vi "4 Edge Rake.vi"(2 "input cluster":errorcluster, 3 "Image Dst Out":T1) -> (0 "B":cluster{sgl, sgl, sgl, sgl}, 1 "M":cluster{sgl, sgl, sgl, sgl})   [LabVIEW 2011]
uses:
  <vilib>/vision/Image Controls.llb/IMAQ Image.ctl
  <vilib>/vision/NI_Vision_Development_Module.lvlib
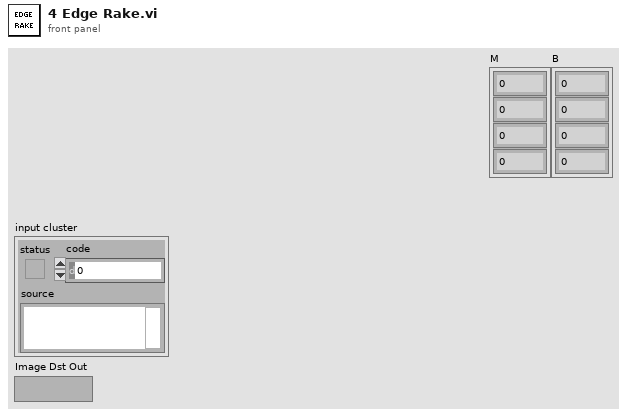
[diagram p1: front panel]
types:
  T1 = typedef "IMAQ Image.ctl" = refnum<image>
  T2 = cluster{"Show Search Area":bool, "Show Search Lines":bool, "Show Edges Found":bool, "Show Result":bool}
  T3 = cluster{"Number of Lines":i32, "Type":enum32{"First Edge Rake", "Best Edge Rake", "Hough Edge Rake", "First Edge Projection", "Best Edge Projection"}, "Min. Score":dbl, "Max. Score":dbl, "Orientation":dbl, "Angle Range":dbl, "Angle Tolerance":dbl, "Step Size":u32, "Min. SNR (db)":dbl, "Min. Points (%)":dbl, "Hough Iterations":i32}
  T4 = cluster{"Edge Polarity":u32, "Kernel Size":u32, "Width":u32, "Minimum Edge Strength":sgl, "Interpolation Type":enum32{"Zero Order", "Bilinear", "Quadratic", "Cubic", "Bilinear Fixed"}, "Data Processing Method":enum32{"Average", "Median"}}
  T5 = cluster{"Global Rectangle":i32[], "Contours":cluster{"ID":enum32{"External", "Internal"}, "Type":u32, "Coordinates":i32[]}[]}
  T6 = cluster{"Point1 (Pixels)":cluster{"X":sgl, "Y":sgl}, "Point2 (Pixels)":cluster{"X":sgl, "Y":sgl}, "Point1 (Real-World)":cluster{"X":sgl, "Y":sgl}, "Point2 (Real-World)":cluster{"X":sgl, "Y":sgl}, "Angle (Pixel)":dbl, "Angle (Real-World)":dbl, "Score":dbl, "Straightness":dbl, "Average SNR (db)":dbl, "Calibration Valid":bool}[]
  T7 = typedef "Search Line.ctl" = cluster{"Start Point":cluster{"X":sgl, "Y":sgl}, "End Point":cluster{"X":sgl, "Y":sgl}, "Edge Info":T8[], "Edge Map":dbl[], "Calibration Valid":bool}
  T8 = typedef "Edge New.ctl" = cluster{"Location (Pixel)":cluster{"X":sgl, "Y":sgl}, "Location (Real-World)":cluster{"X":sgl, "Y":sgl}, "Distance (Pixel)":dbl, "Distance (Real-World)":dbl, "Strength":dbl, "Noise":dbl, "Rising?":bool}
  T9 = cluster{"Straight Edges":cluster{"Point1 (Pixels)":cluster{"X":sgl, "Y":sgl}, "Point2 (Pixels)":cluster{"X":sgl, "Y":sgl}, "Point1 (Real-World)":cluster{"X":sgl, "Y":sgl}, "Point2 (Real-World)":cluster{"X":sgl, "Y":sgl}, "Angle (Pixel)":dbl, "Angle (Real-World)":dbl, "Score":dbl, "Straightness":dbl, "Average SNR (db)":dbl, "Calibration Valid":bool}[], "Search Lines Information":T7[], "Used Edges":cluster{"Edge Information":T8[]}[]}
  T10 = cluster{"Point1 (Pixels)":cluster{"X":sgl, "Y":sgl}, "Point2 (Pixels)":cluster{"X":sgl, "Y":sgl}, "Point1 (Real-World)":cluster{"X":sgl, "Y":sgl}, "Point2 (Real-World)":cluster{"X":sgl, "Y":sgl}, "Angle (Pixel)":dbl, "Angle (Real-World)":dbl, "Score":dbl, "Straightness":dbl, "Average SNR (db)":dbl, "Calibration Valid":bool}
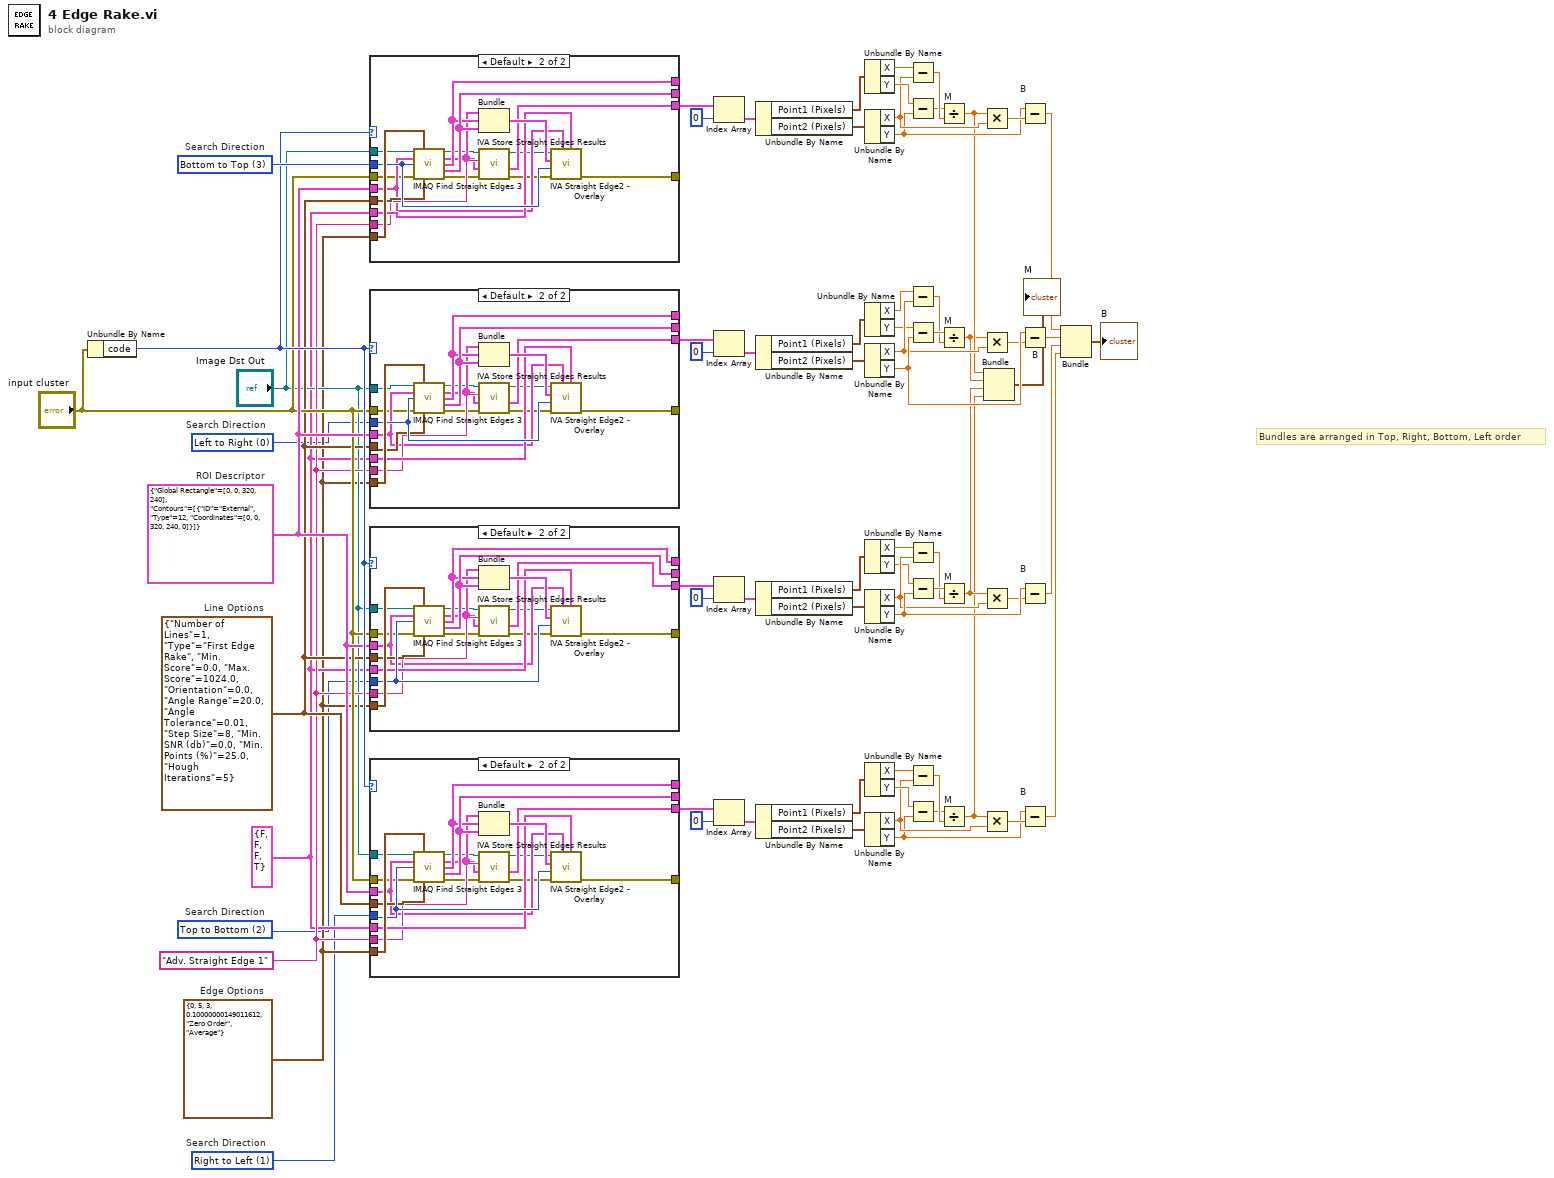
[diagram p0: block diagram]
diagram:
  w54 = u32 1 items=["Left to Right", "Right to Left", "Top to Bottom", "Bottom to Top"]  # Search Direction
  w56 = u32 2 items=["Left to Right", "Right to Left", "Top to Bottom", "Bottom to Top"]  # Search Direction
  w55 = u32 0 items=["Left to Right", "Right to Left", "Top to Bottom", "Bottom to Top"]  # Search Direction
  w60 = "Adv. Straight Edge 1" ("Step Name")
  w58 = T2 {"Show Search Area"=FALSE, "Show Search Lines"=FALSE, "Show Edges Found"=FALSE, "Show Result"=TRUE} ("Setup")
  w61 = T3 {"Number of Lines"=1, "Type"=enum."First Edge Rake", "Min. Score"=0.0, "Max. Score"=1024.0, "Orientation"=0.0, "Angle Range"=20.0, "Angle Tolerance"=0.01, "Step Size"=8, "Min. SNR (db)"=0.0, "Min. Points (%)"=25.0, "Hough Iterations"=5}  # Line Options
  w70 = u32 3 items=["Left to Right", "Right to Left", "Top to Bottom", "Bottom to Top"]  # Search Direction
  w57 = T4 {"Edge Polarity"=0, "Kernel Size"=5, "Width"=3, "Minimum Edge Strength"=0.1, "Interpolation Type"=enum."Zero Order", "Data Processing Method"=enum."Average"}  # Edge Options
  w63 = T5 {"Global Rectangle"=[0, 0, 320, 240], "Contours"=[{"ID"=enum."External", "Type"=12, "Coordinates"=[0, 0, 320, 240, 0]}]}  # ROI Descriptor
  # "Bundles are arranged in Top, Right, Bottom, Left order"
  n1 = Unbundle By Name("input cluster") -> ("code"=w64:i32)
  n2 = case shown="Default" w64 {
    tunnel: w57 -> [_ w88]
    tunnel: w70 -> [_ w87]
    tunnel: w61 -> [_ w86]
    tunnel: [_ w84] -> _
    tunnel: w58 -> [_ w83]
    tunnel: [_ w82] -> _
    tunnel: [_ w81] -> _
    tunnel: w60 -> [_ w80]
    tunnel: [_ w79] -> w65
    tunnel: w63 -> [_ w77]
    tunnel: "input cluster" -> [_ w72]
    tunnel: "Image Dst Out" -> [_ w71]
    frame -1074396199, -1074396198 {
      # "Discard Coordinate System Error"
    }
    frame Default {
      n3 = call "IMAQ Find Straight Edges 3"("Image"=w71, "Edge Options"=w88, "ROI Descriptor"=w77, "Search Direction"=w87, "error in (no error)"=w72, "Line Options"=w86) -> ("Image (duplicate)"=w76:T1, "Straight Edges"=w78:T6, "Search Lines Information"=w81:T7[], "Used Edges"=w82:cluster{"Edge Information":T8[]}[], "error out"=w74:errorcluster)  [unwired: 1 in, 4 out]
      n4 = Bundle("Straight Edges"=w78, "Search Lines Information"=w81, "Used Edges"=w82) -> (w85:T9)  [unwired: 1 out]
      n5 = call <vilib>:"IVA Store Straight Edges Results.vi"("error in (no error)"=w74, "Straight Edges"=w78, "Step Name"=w80, "Image in"=w76) -> ("error out"=w73:errorcluster, "Straight Edges dup"=w79:T6, "Image dup"=w75:T1)  [unwired: 5 out]
      n6 = call <vilib>:"IVA Straight Edge2 - Overlay.vi"("Setup"=w83, "Search Area"=w77, "error in (no error)"=w73, "Scan Direction"=w87, "Edge Results"=w85, "Image In"=w75) -> ("error out"=w84:errorcluster)  [unwired: 1 in, 4 out]
    }
  }
  n7 = case shown="Default" w64 {
    tunnel: w57 -> [_ w106]
    tunnel: w55 -> [_ w105]
    tunnel: w61 -> [_ w104]
    tunnel: [_ w102] -> _
    tunnel: w58 -> [_ w101]
    tunnel: [_ w100] -> _
    tunnel: [_ w99] -> _
    tunnel: w60 -> [_ w98]
    tunnel: [_ w97] -> w11
    tunnel: w63 -> [_ w95]
    tunnel: "input cluster" -> [_ w90]
    tunnel: "Image Dst Out" -> [_ w89]
    frame -1074396199, -1074396198 {
      # "Discard Coordinate System Error"
    }
    frame Default {
      n8 = call "IMAQ Find Straight Edges 3"("Image"=w89, "Edge Options"=w106, "ROI Descriptor"=w95, "Search Direction"=w105, "error in (no error)"=w90, "Line Options"=w104) -> ("Image (duplicate)"=w94:T1, "Straight Edges"=w96:T6, "Search Lines Information"=w99:T7[], "Used Edges"=w100:cluster{"Edge Information":T8[]}[], "error out"=w92:errorcluster)  [unwired: 1 in, 4 out]
      n9 = Bundle("Straight Edges"=w96, "Search Lines Information"=w99, "Used Edges"=w100) -> (w103:T9)  [unwired: 1 out]
      n10 = call <vilib>:"IVA Store Straight Edges Results.vi"("error in (no error)"=w92, "Straight Edges"=w96, "Step Name"=w98, "Image in"=w94) -> ("error out"=w91:errorcluster, "Straight Edges dup"=w97:T6, "Image dup"=w93:T1)  [unwired: 5 out]
      n11 = call <vilib>:"IVA Straight Edge2 - Overlay.vi"("Setup"=w101, "Search Area"=w95, "error in (no error)"=w91, "Scan Direction"=w105, "Edge Results"=w103, "Image In"=w93) -> ("error out"=w102:errorcluster)  [unwired: 1 in, 4 out]
    }
  }
  n12 = case shown="Default" w64 {
    tunnel: w57 -> [_ w124]
    tunnel: w56 -> [_ w123]
    tunnel: w61 -> [_ w122]
    tunnel: [_ w120] -> _
    tunnel: w58 -> [_ w119]
    tunnel: [_ w118] -> _
    tunnel: [_ w117] -> _
    tunnel: w60 -> [_ w116]
    tunnel: [_ w115] -> w13
    tunnel: w63 -> [_ w113]
    tunnel: "input cluster" -> [_ w108]
    tunnel: "Image Dst Out" -> [_ w107]
    frame -1074396199, -1074396198 {
      # "Discard Coordinate System Error"
    }
    frame Default {
      n13 = call "IMAQ Find Straight Edges 3"("Image"=w107, "Edge Options"=w124, "ROI Descriptor"=w113, "Search Direction"=w123, "error in (no error)"=w108, "Line Options"=w122) -> ("Image (duplicate)"=w112:T1, "Straight Edges"=w114:T6, "Search Lines Information"=w117:T7[], "Used Edges"=w118:cluster{"Edge Information":T8[]}[], "error out"=w110:errorcluster)  [unwired: 1 in, 4 out]
      n14 = Bundle("Straight Edges"=w114, "Search Lines Information"=w117, "Used Edges"=w118) -> (w121:T9)  [unwired: 1 out]
      n15 = call <vilib>:"IVA Store Straight Edges Results.vi"("error in (no error)"=w110, "Straight Edges"=w114, "Step Name"=w116, "Image in"=w112) -> ("error out"=w109:errorcluster, "Straight Edges dup"=w115:T6, "Image dup"=w111:T1)  [unwired: 5 out]
      n16 = call <vilib>:"IVA Straight Edge2 - Overlay.vi"("Setup"=w119, "Search Area"=w113, "error in (no error)"=w109, "Scan Direction"=w123, "Edge Results"=w121, "Image In"=w111) -> ("error out"=w120:errorcluster)  [unwired: 1 in, 4 out]
    }
  }
  n17 = case shown="Default" w64 {
    tunnel: w57 -> [_ w142]
    tunnel: w54 -> [_ w141]
    tunnel: w61 -> [_ w140]
    tunnel: [_ w138] -> _
    tunnel: w58 -> [_ w137]
    tunnel: [_ w136] -> _
    tunnel: [_ w135] -> _
    tunnel: w60 -> [_ w134]
    tunnel: [_ w133] -> w12
    tunnel: w63 -> [_ w131]
    tunnel: "input cluster" -> [_ w126]
    tunnel: "Image Dst Out" -> [_ w125]
    frame -1074396199, -1074396198 {
      # "Discard Coordinate System Error"
    }
    frame Default {
      n18 = call "IMAQ Find Straight Edges 3"("Image"=w125, "Edge Options"=w142, "ROI Descriptor"=w131, "Search Direction"=w141, "error in (no error)"=w126, "Line Options"=w140) -> ("Image (duplicate)"=w130:T1, "Straight Edges"=w132:T6, "Search Lines Information"=w135:T7[], "Used Edges"=w136:cluster{"Edge Information":T8[]}[], "error out"=w128:errorcluster)  [unwired: 1 in, 4 out]
      n19 = Bundle("Straight Edges"=w132, "Search Lines Information"=w135, "Used Edges"=w136) -> (w139:T9)  [unwired: 1 out]
      n20 = call <vilib>:"IVA Store Straight Edges Results.vi"("error in (no error)"=w128, "Straight Edges"=w132, "Step Name"=w134, "Image in"=w130) -> ("error out"=w127:errorcluster, "Straight Edges dup"=w133:T6, "Image dup"=w129:T1)  [unwired: 5 out]
      n21 = call <vilib>:"IVA Straight Edge2 - Overlay.vi"("Setup"=w137, "Search Area"=w131, "error in (no error)"=w127, "Scan Direction"=w141, "Edge Results"=w139, "Image In"=w129) -> ("error out"=w138:errorcluster)  [unwired: 1 in, 4 out]
    }
  }
  n22 = Index Array(array=w65, index=0) -> (element=w68:T10)
  n23 = Index Array(array=w11, index=0) -> (element=w37:T10)
  n24 = Index Array(array=w13, index=0) -> (element=w15:T10)
  n25 = Index Array(array=w12, index=0) -> (element=w34:T10)
  n26 = Unbundle By Name(w68) -> ("Point1 (Pixels)"=w67:cluster{"X":sgl, "Y":sgl}, "Point2 (Pixels)"=w66:cluster{"X":sgl, "Y":sgl})
  n27 = Unbundle By Name(w37) -> ("Point1 (Pixels)"=w38:cluster{"X":sgl, "Y":sgl}, "Point2 (Pixels)"=w39:cluster{"X":sgl, "Y":sgl})
  n28 = Unbundle By Name(w15) -> ("Point1 (Pixels)"=w16:cluster{"X":sgl, "Y":sgl}, "Point2 (Pixels)"=w17:cluster{"X":sgl, "Y":sgl})
  n29 = Unbundle By Name(w34) -> ("Point1 (Pixels)"=w33:cluster{"X":sgl, "Y":sgl}, "Point2 (Pixels)"=w32:cluster{"X":sgl, "Y":sgl})
  n30 = Unbundle By Name(w67) -> ("X"=w51:sgl, "Y"=w52:sgl)
  n31 = Unbundle By Name(w66) -> ("X"=w49:sgl, "Y"=w47:sgl)
  n32 = Unbundle By Name(w38) -> ("X"=w42:sgl, "Y"=w41:sgl)
  n33 = Unbundle By Name(w39) -> ("X"=w44:sgl, "Y"=w46:sgl)
  n34 = Unbundle By Name(w16) -> ("X"=w20:sgl, "Y"=w19:sgl)
  n35 = Unbundle By Name(w17) -> ("X"=w22:sgl, "Y"=w24:sgl)
  n36 = Unbundle By Name(w33) -> ("X"=w29:sgl, "Y"=w30:sgl)
  n37 = Unbundle By Name(w32) -> ("X"=w27:sgl, "Y"=w25:sgl)
  n38 = Subtract(x=w51, y=w49) -> (x-y=w53:sgl)
  n39 = Subtract(x=w52, y=w47) -> (x-y=w50:sgl)
  n40 = Subtract(x=w42, y=w44) -> (x-y=w40:sgl)
  n41 = Subtract(x=w41, y=w46) -> (x-y=w43:sgl)
  n42 = Subtract(x=w20, y=w22) -> (x-y=w18:sgl)
  n43 = Subtract(x=w19, y=w24) -> (x-y=w21:sgl)
  n44 = Subtract(x=w29, y=w27) -> (x-y=w31:sgl)
  n45 = Subtract(x=w30, y=w25) -> (x-y=w28:sgl)
  n46 = Divide "M"(x=w50, y=w53) -> (x/y=w10:sgl)
  n47 = Divide "M"(x=w43, y=w40) -> (x/y=w8:sgl)
  n48 = Divide "M"(x=w21, y=w18) -> (x/y=w6:sgl)
  n49 = Divide "M"(x=w28, y=w31) -> (x/y=w3:sgl)
  n50 = Multiply(x=w10, y=w49) -> (x*y=w48:sgl)
  n51 = Multiply(x=w8, y=w44) -> (x*y=w45:sgl)
  n52 = Multiply(x=w6, y=w22) -> (x*y=w23:sgl)
  n53 = Multiply(x=w3, y=w27) -> (x*y=w26:sgl)
  n54 = Bundle(w10, w8, w6, w3) -> (→"M":cluster{sgl, sgl, sgl, sgl})  [unwired: 1 in]
  n55 = Subtract "B"(x=w47, y=w48) -> (x-y=w9:sgl)
  n56 = Subtract "B"(x=w46, y=w45) -> (x-y=w7:sgl)
  n57 = Subtract "B"(x=w24, y=w23) -> (x-y=w5:sgl)
  n58 = Subtract "B"(x=w25, y=w26) -> (x-y=w4:sgl)
  n59 = Bundle(w9, w7, w5, w4) -> (→"B":cluster{sgl, sgl, sgl, sgl})  [unwired: 1 in]
